vi "Initialize.vi"(0 "VISA resource name":refnum<visa-resource-name>, 5 "Serial Configuration":T1={"Baud Rate"=115200, "Parity"=0, "Data Bits"=8, "Stop Bits"=10, "Flow Control"=0} {"Flow Control" items=["None", "XON/XOFF", "RTS/CTS", "XON/XOFF & RTS/CTS", "DTR/DSR", "XON/XOFF & DTR/DSR"]; "Stop Bits" items=["1.0"=10, "1.5"=15, "2.0"=20]; "Data Bits" items=["7"=7, "8"=8]; "Parity" items=["None", "Odd", "Even", "Mark", "Space"]; "Baud Rate" items=["300"=300, "600"=600, "1200"=1200, "2400"=2400, "4800"=4800, "9600"=9600, "19200"=19200, "38400"=38400, "115200"=115200]}, 9 "Reset (True)":bool=TRUE, 11 "error in (no error)":errorcluster, 12 "Timeout (10000 ms)":u32=10000) -> (4 "VISA resource name out":refnum<visa-resource-name>, 15 "error out":errorcluster)   [LabVIEW 2014, in "Associated Power Technologies 8500 Series.lvlib"]
doc: "Establishes communication with the instrument and optionally performs an instrument identification query and/or an instrument reset. It also places the instrument in a default state needed for other instrument driver operations. Therefore, call this VI before calling other instrument driver VIs for this instrument. Generally, you need to call the Initialize VI only once at the beginning of an application."
uses:
  <instrlib>/Associated Power Technologies 8500 Series/Associated Power Technologies 8500 Series.lvlib
  <instrlib>/Associated Power Technologies 8500 Series/Private/Extended User Data.ctl
panel:
  # "(c) 2020 Associated Power Technologies.  ALL RIGHTS RESERVED."
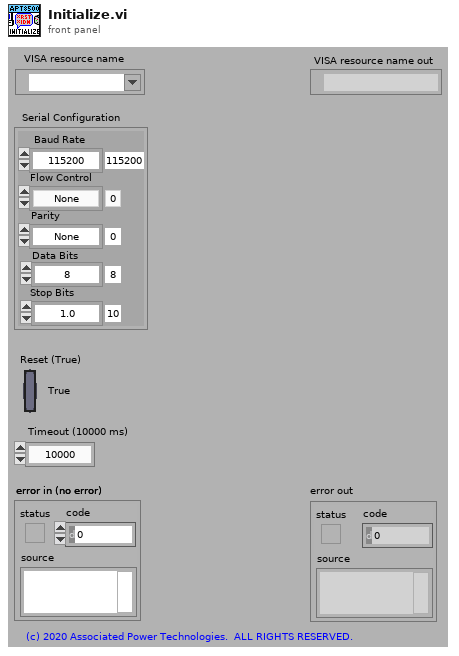
[diagram p1: front panel]
types:
  T1 = cluster{"Baud Rate":u32, "Parity":u16, "Data Bits":u16, "Stop Bits":u16, "Flow Control":u16}
  T2 = typedef "Associated Power Technologies 8500 Series.lvlib/Extended User Data.ctl" = cluster{"Firmware Version":string, "APT Models":enum16{"APT-8505", "APT-8512", "APT-8520", "APT-8540"}}
  T3 = enum16{"APT-8505", "APT-8512", "APT-8520", "APT-8540"}
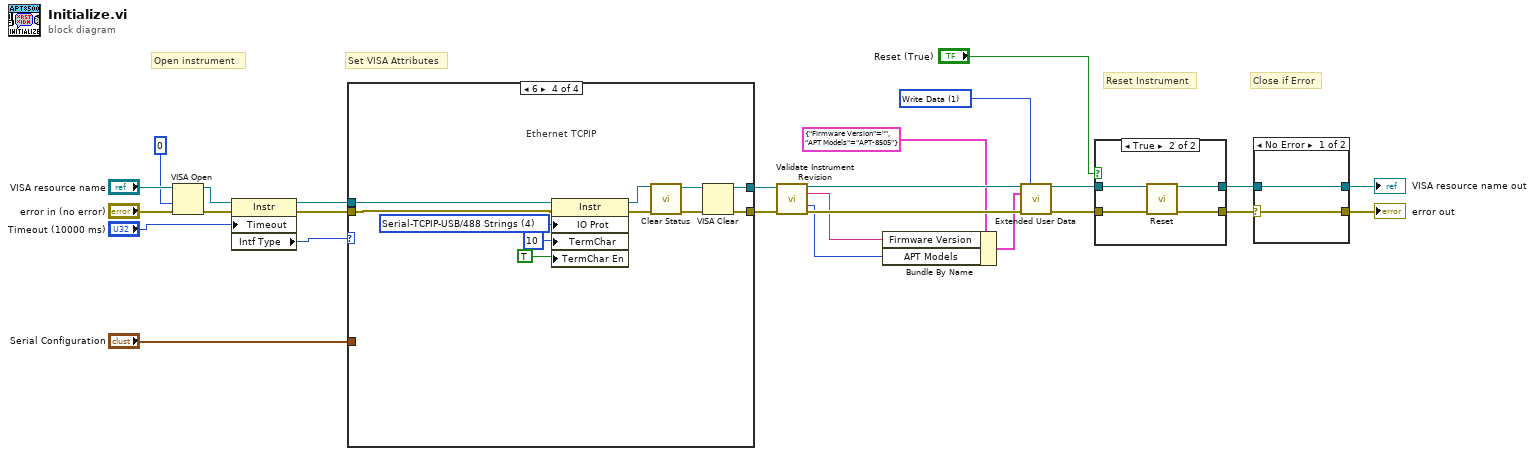
[diagram p0: block diagram]
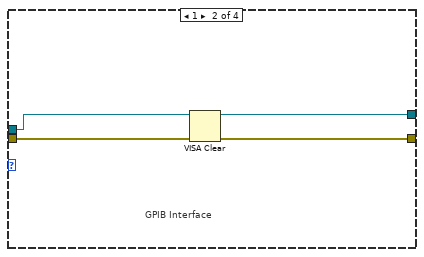
[diagram p3: hidden frame]
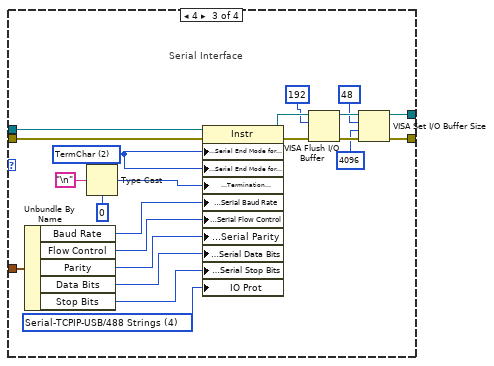
[diagram p4: hidden frame]
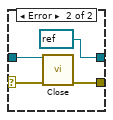
[diagram p5: hidden frame]
diagram:
  w12 = u16 1 items=["Read Data", "Write Data", "Clear Data", "Clear ALL Data"] ("Action")
  # "Set VISA Attributes"
  # "Close if Error"
  # "Reset Instrument"
  # "Open instrument"
  n1 = VISA Open(access mode=u32 0, error in (no error)="error in (no error)", VISA resource name="VISA resource name") -> (VISA resource name=w21:refnum<visa-resource-name>, error out=w20:errorcluster)  [unwired: 2 in]
  n2 = property on="Property Node" class="Instr"(reference=w21, error in=w20, "Timeout"="Timeout (10000 ms)") -> (reference out=w11:refnum<visa-resource-name>, error out=w10:errorcluster, "Intf Type"=w9:u16)
  n3 = case shown="6" w9 {
    tunnel: [w28 w31 w54 w57] -> w23
    tunnel: [w27 w32 w52 w56] -> w22
    tunnel: w11 -> [w28 w29 w34 w65]
    tunnel: w10 -> [w27 w30 w33 w61]
    tunnel: "Serial Configuration" -> [_ _ w41 _]
    frame Default {
    }
    frame 1 {
      # "GPIB Interface"
      n4 = VISA Clear(VISA resource name=w29, error in (no error)=w30) -> (VISA resource name out=w31:refnum<visa-resource-name>, error out=w32:errorcluster)
    }
    frame 4 {
      w35 = u16 4 items=["Normal"=1, "VXI/FDC"=2, "GPIB/HS488"=3, "Serial-TCPIP-USB/488 Strings"=4, "USBTMC/Vendor-Specific"=5] ("Message Based Settings:IO Protocol")
      w48 = u16 2 items=["None", "LastBit", "TermChar"] ("Serial Settings:Serial End Mode for Reads")
      # "Serial Interface"
      n5 = Unbundle By Name(w41) -> ("Baud Rate"=w46:u32, "Flow Control"=w43:u16, "Parity"=w44:u16, "Data Bits"=w45:u16, "Stop Bits"=w42:u16)
      n6 = Type Cast(type=u8 0, x="\n" ("Line Feed Constant")) -> (*(type *) &x=w47:u8)
      n7 = property on="Property Node" class="Instr"(reference=w34, error in=w33, "Serial Settings:Serial End Mode for Reads"=w48, "Serial Settings:Serial End Mode for Writes"=w48, "Message Based Settings:Termination Character"=w47, "Serial Settings:Serial Baud Rate"=w46, "Serial Settings:Serial Flow Control"=w43, "Serial Settings:Serial Parity"=w44, "Serial Settings:Serial Data Bits"=w45, "Serial Settings:Serial Stop Bits"=w42, "IO Prot"=w35) -> (reference out=w51:refnum<visa-resource-name>, error out=w53:errorcluster)
      n8 = VISA Flush I/O Buffer(VISA resource name=w51, mask (16)=u16 192, error in (no error)=w53) -> (VISA resource name out=w40:refnum<visa-resource-name>, error out=w39:errorcluster)
      n9 = VISA Set I/O Buffer Size(VISA resource name=w40, mask (16)=u16 48, size (4096)=u32 4096 ("size (0)"), error in (no error)=w39) -> (VISA resource name out=w54:refnum<visa-resource-name>, error out=w52:errorcluster)
    }
    frame 6 {
      w64 = u16 4 items=["Normal"=1, "VXI/FDC"=2, "GPIB/HS488"=3, "Serial-TCPIP-USB/488 Strings"=4, "USBTMC/Vendor-Specific"=5] ("Message Based Settings:IO Protocol")
      # "Ethernet TCPIP"
      n10 = property on="Property Node" class="Instr"(reference=w65, error in=w61, "IO Prot"=w64, "TermChar"=u8 10 ("Message Based Settings:Termination Character"), "TermChar En"=TRUE ("Message Based Settings:Termination Character Enable")) -> (reference out=w59:refnum<visa-resource-name>, error out=w60:errorcluster)
      n11 = call <instrlib>:"Clear Status.vi"("VISA resource name"=w59, "error in (no error)"=w60) -> ("VISA resource name out"=w55:refnum<visa-resource-name>, "error out"=w58:errorcluster)  [unwired: 12 in]
      n12 = VISA Clear(VISA resource name=w55, error in (no error)=w58) -> (VISA resource name out=w57:refnum<visa-resource-name>, error out=w56:errorcluster)
    }
  }
  n13 = call <instrlib>:"Validate Instrument Revision.vi"("VISA resource name"=w23, "error in (no error)"=w22) -> ("VISA resource name out"=w8:refnum<visa-resource-name>, "Firmware Version"=w3:string, "Model Number"=w4:T3, "error out"=w7:errorcluster)  [unwired: 10 in]
  n14 = Bundle By Name(cluster=T2 {"Firmware Version"="", "APT Models"=enum."APT-8505"} ("User Data In"), "Firmware Version"=w3, "APT Models"=w4) -> (w6:T2)
  n15 = call <instrlib>:"Extended User Data.vi"("VISA resource name"=w8, "Action"=w12, "User Data In"=w6, "Error In (no error)"=w7) -> ("VISA resource name out"=w14:refnum<visa-resource-name>, "Error Out"=w13:errorcluster)  [unwired: 9 in, 1 out]
  n16 = case shown="True" "Reset (True)" {
    tunnel: w13 -> [w66 w68]
    tunnel: [w66 w70] -> w2
    tunnel: w14 -> [w67 w69]
    tunnel: [w67 w71] -> w17
    frame False {
    }
    frame True {
      n17 = call <instrlib>:"Reset.vi"("VISA resource name"=w69, "error in (no error)"=w68) -> ("VISA resource name out"=w71:refnum<visa-resource-name>, "error out"=w70:errorcluster)  [unwired: 12 in]
    }
  }
  n18 = case shown="No Error" w2 {
    selector: w2 -> [w72 w75]
    tunnel: w17 -> [w73 w76]
    tunnel: [w73 refnum<visa-resource-name> refnum ("VISA resource name out")] -> w19
    tunnel: [w72 w77] -> w18
    frame No Error {
    }
    frame Error {
      n19 = call <instrlib>:"Close.vi"("VISA resource name"=w76, "error in (no error)"=w75) -> ("error out"=w77:errorcluster)  [unwired: 13 in]
    }
  }
  "VISA resource name out" <- w19
  "error out" <- w18
